vi "ControlApp.vi"() -> ()   [LabVIEW 2022 SP3]
uses:
  <vilib>/DAQmx/create/channels.llb/DAQmx Create Channel (AI-Voltage-Basic).vi
  <vilib>/DAQmx/create/channels.llb/DAQmx Create Channel (AO-Voltage-Basic).vi
  <vilib>/DAQmx/read.llb/DAQmx Read (Analog DBL 1Chan 1Samp).vi
  <vilib>/DAQmx/write.llb/DAQmx Write (Analog DBL 1Chan 1Samp).vi
  <vilib>/Simulation/Implementation/XNodeFramework/SimXNode/SimX.xnode
  SubVIs/Air Heater Model.vi
  <vilib>/Simulation/Implementation/Shared/SIMSCR Execution Mode.ctl
  <vilib>/Simulation/Scripting/Companion Diagram/SimConfigNode/_simSolvers.ctl
  <vilib>/Simulation/Scripting/Companion Diagram/SimConfigNode/SimParams.ctl
  <vilib>/Simulation/Scripting/Companion Diagram/SimConfigNode/SimDog.xnode
  <vilib>/OPCUA/controls/Write Status.ctl
  <vilib>/OPCUA/controls/NodeId.ctl
  <vilib>/OPCUA/client/Multiple Write Double.vi
  <vilib>/OPCUA/controls/OPC UA Client Refnum.ctl
panel:
  out "Status":bool
  out "OPC UA Client Reference":T1="tOPCUAClient3"
  out "Temperature":dbl=25.00772115553251 caption="Temperature [C]:" format="%.2g"
  out "Current Time":string="2018-10-12 13:37:48"
  out "Database Connection":refnum<k7>
  out "Error Out":errorcluster
  in  "Error In":errorcluster
  in  "Stop Button":bool
  in  "Start Button":bool
  in  "Tab Control":T2(tab)
  out "Measurement Chart":cluster{"Tout [C]":dbl, "Setpoint [C]":dbl}(graph)={"Tout [C]"=25.00772115553251, "Setpoint [C]"=25.0}
  out "Control Chart":dbl(graph)=1.0759899998167255
  in  "Process Type":enum16{"Model", "Real Process"}(ring)
  in  "Manual Control Signal [V]":dbl min=0.0 max=5.0 step=0.1 format="%.1g"
  in  "Auto?":bool=TRUE
  in  "Setpoint [C]":dbl(slide)=25.0 scale=20.0..50.0
  in  "PID Parameters":cluster{"Kp":dbl, "Ti [s]":dbl, "Td [s]":dbl}={"Kp"=0.55, "Ti [s]"=18.0, "Td [s]"=0.0}
  in  "Write to File":bool
  in  "File Path":path=path "C:/Temp/MeasurementData.lvm"
  in  "Write to SQL Server":bool
  in  "OPC Settings":T3={"OPC Server Endpoint URL"="opc.tcp://XPS15HPH:49580", "OPC Node Id"="ns=2;s=ProcessData.Temperature"}
  in  "Database":T4={"Data Source Name"="XPS15HPH\\SQLEXPRESS", "Database Name"="MEASUREMENTS", "User Name"="sa", "Password"="ullabella"} caption="Database Connection:"
  in  "DAQ Settings":T5={"Analog Input Channel"="Dev1/ai0", "AImin[V]"=1, "AImax[V]"=5, "Analog Output Channel"="Dev1/ao0", "AOmin[V]"=0, "AOmax[V]"=5} {"AOmax[V]" min=-10 max=10 step=1; "AOmin[V]" min=-10 max=10 step=1; "AImax[V]" min=-10 max=10 step=1; "AImin[V]" min=-10 max=10 step=1}
  out "Error Message":errorcluster
  in  "Exit Button":bool
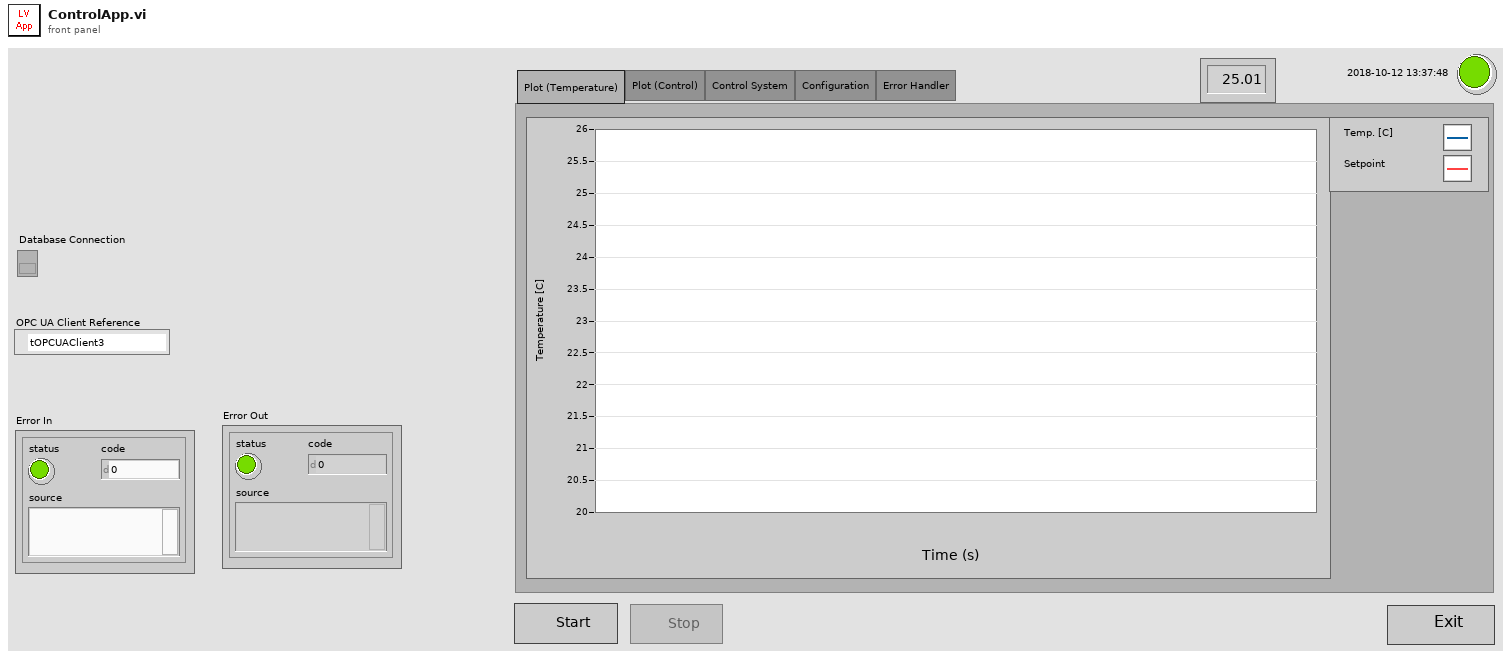
[diagram p1: front panel]
types:
  T1 = typedef "OPC UA Client Refnum.ctl" = refnum<k21>
  T2 = enum32{"Plot (Temperature)", "Plot (Control)", "Control System", "Configuration", "Error Handler", "Cloud Service"}
  T3 = cluster{"OPC Server Endpoint URL":string, "OPC Node Id":string}
  T4 = cluster{"Data Source Name":string, "Database Name":string, "User Name":string, "Password":string}
  T5 = cluster{"Analog Input Channel":tag, "AImin[V]":i32, "AImax[V]":i32, "Analog Output Channel":tag, "AOmin[V]":i32, "AOmax[V]":i32}
  T6 = enum8{"Enabled", "Disabled", "Disabled and Grayed Out"}
  T7 = enum16{"Simulate to Completion", "Single Time-Step Simulation (Fixed Step Only)"}
  T8 = typedef "SimParams.ctl" = cluster{"Initial Time (s)":dbl, "Final Time (s)":dbl, "Step Size (s)":dbl, "ODE Solver":T9, "Minimum Step Size (s)":dbl, "Maximum Step Size (s)":dbl, "Relative Tolerance":dbl, "Absolute Tolerance":dbl, "Software Timing":bool, "Initial Step Size (s)":dbl, "Automatic Fixed Step Size?":bool, "Automatic Discrete Step Size?":bool, "Discrete Step Size (s)":dbl, "Calculate using Time Step":bool, "Solver Wired?":bool, "Prev.Frm.Expected End":u64, "Prev.Frm.Actual End":u64, "Prev.Frm.Finished Late?":bool, "Prev.Iter.Expected End":u64, "Prev.Iter.Actual End":u64, "Prev.Iter.Finished Late?":bool, "Expected Iteration Start":u64, "Actual Iteration Start":u64, "Expected Frame Start":u64, "Actual Frame Start":u64, "Source Name":string, "Name":string, "Period":i64, "Deadline":i64, "Offset":i64, "Start":i64, "Priority":i32, "Timeout":i32, "Processor":i32, "Mode":enum32{"No Change", "Process missed periods, maintain original phase", "Discard missed periods, maintain original phase", "Process missed periods, ignore original phase", "Discard missed periods, ignore original phase"}, "Wakeup reason":enum32{"Normal", "Aborted", "Asynchronous wakeup", "Timing source error", "Timed loop error", "Timeout"}, "Error":errorcluster, "Source Type":string, "Secondary Source Type":string, "Global End Time":u64, "Global Start Time":u64, "Full Solver Reset":bool, "Execution Mode":T10, "Nan/Inf Check":bool, "Custom Solver Library":string, "Solver Is Variable":bool, "custom solver name":string, "Signal Collection Decimation":u32}
  T9 = typedef "_simSolvers.ctl" = enum16{"Runge-Kutta 1 (Euler)", "Runge-Kutta 2", "Runge-Kutta 3", "Runge-Kutta 4", "Runge-Kutta 23 (variable)", "Runge-Kutta 45 (variable)", "BDF (variable)", "Adams-Moulton (variable)", "Rosenbrock (variable)", "Discrete States Only", "SDIRK 4 (variable)", "Radau 5 (variable)", "Radau 9 (variable)", "Radau 13 (variable)", "Radau [Variable Order] (variable)", "Gear's Method (variable)", "Linearizer", "State Query", "Trim Eval", "Custom Solver"}
  T10 = typedef "SIMSCR Execution Mode.ctl" = enum16{"Simulate to Completion", "Single Time-Step Simulation (Fixed Step Only)"}
  T11 = cluster{"message mode":enum16{"None", "Sign", "Sign and Encrypt"}, "security":enum16{"Basic256", "Basic128Rsa15"}}
  T12 = cluster{"Vmin":dbl, "Vmax":dbl, "EUmin":dbl, "EUmax":dbl}
  T13 = typedef "NodeId.ctl" = string
  T14 = typedef "Write Status.ctl" = u32
  T15 = cluster{"node ID":T13, "value":dbl, "timestamp (current time)":timestamp, "node status":T14}
  T16 = cluster{"node ID":T13, "value":dbl, "timestamp (current time)":timestamp, "node status":T14}[]
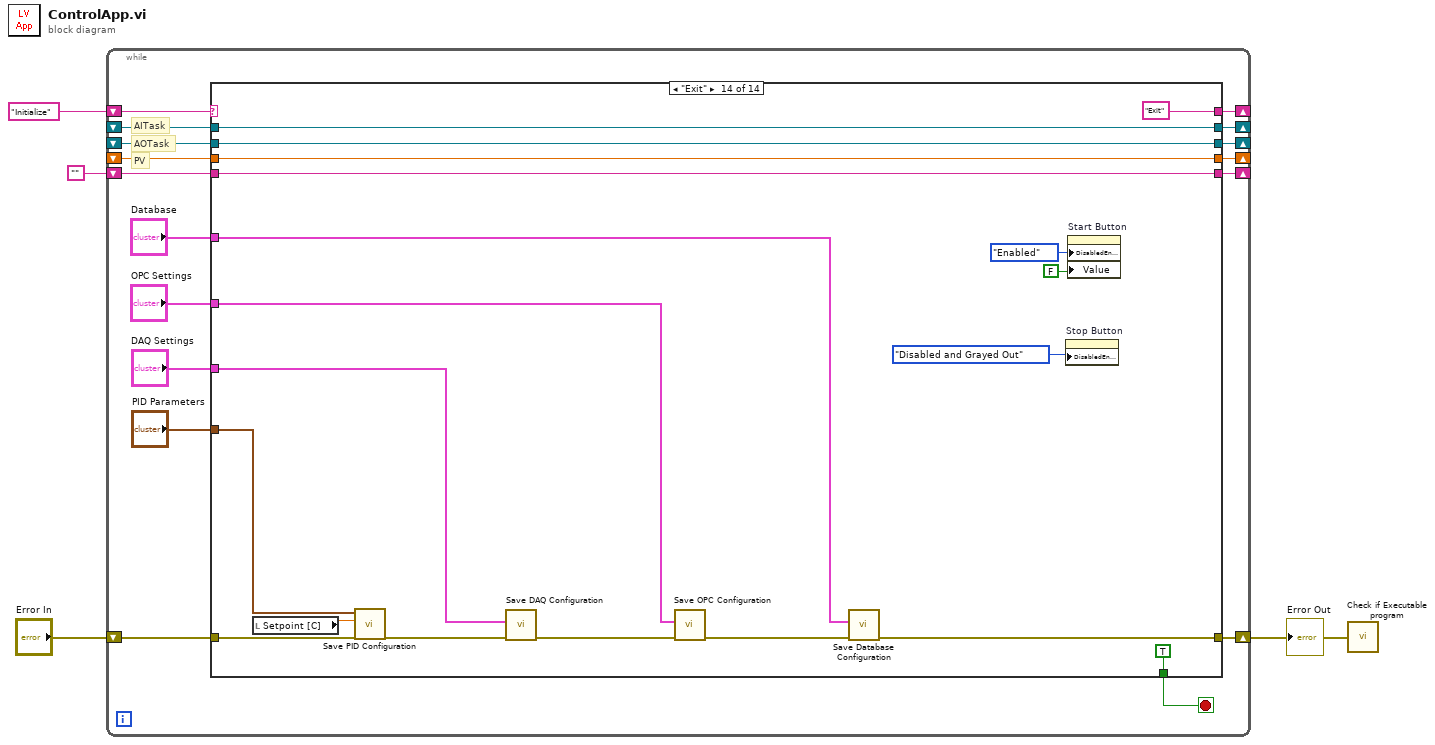
[diagram p0: block diagram]
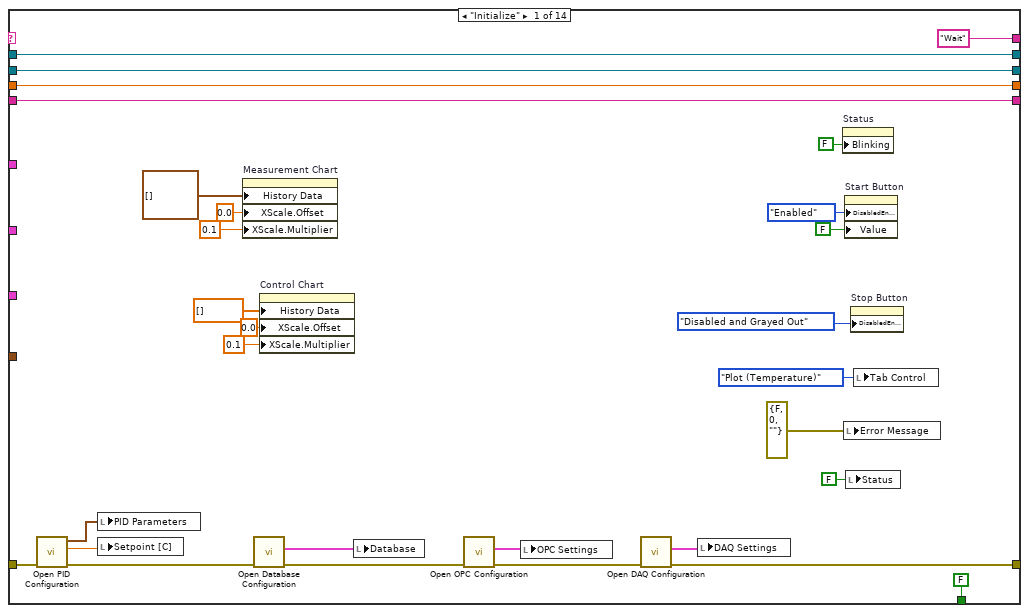
[diagram p2: hidden frame]
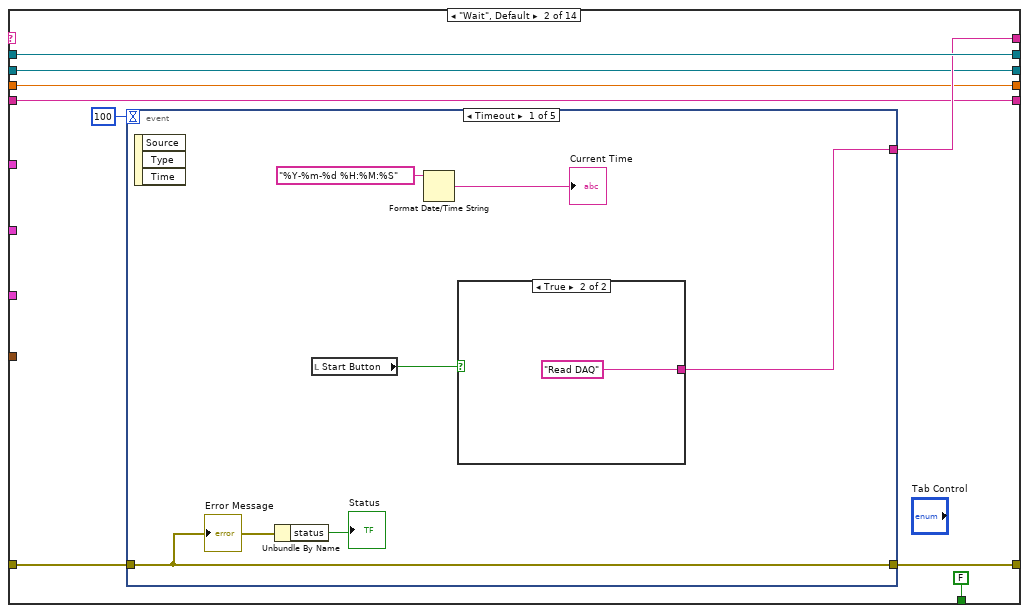
[diagram p3: hidden frame]
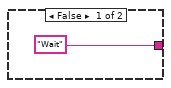
[diagram p4: hidden frame]
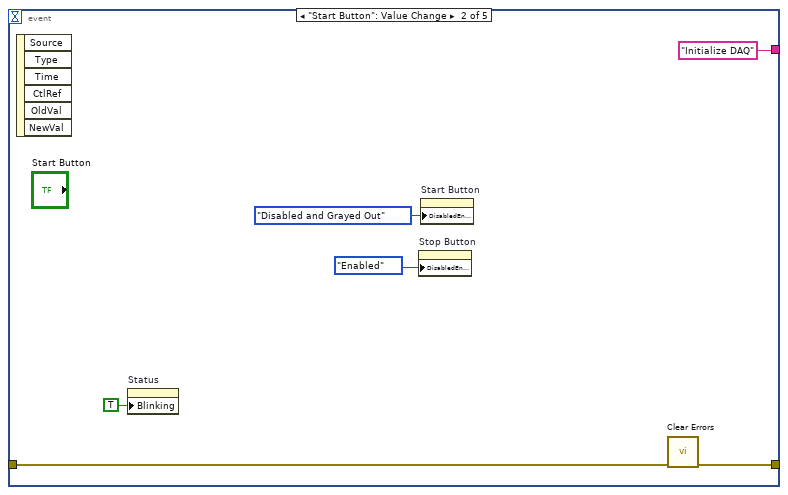
[diagram p5: hidden frame]
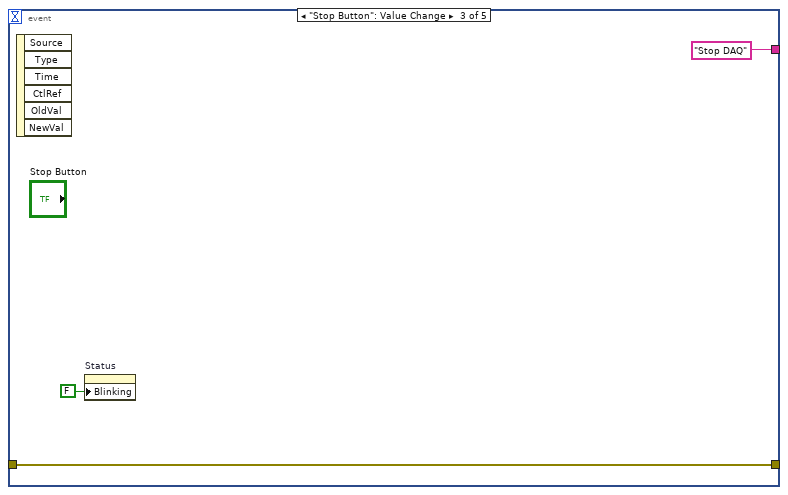
[diagram p6: hidden frame]
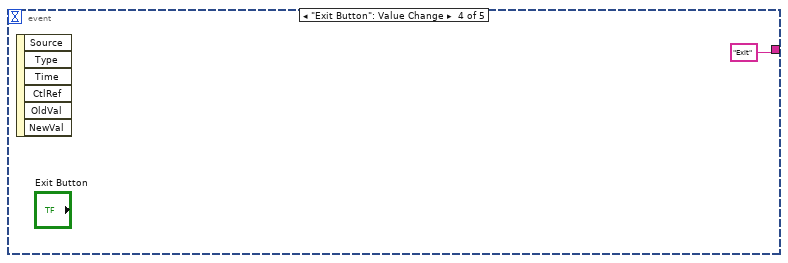
[diagram p7: hidden frame]
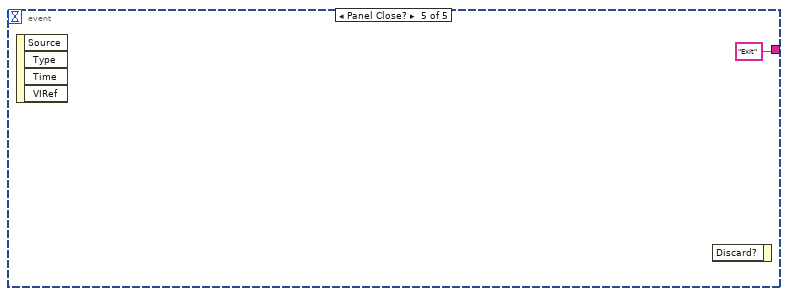
[diagram p8: hidden frame]
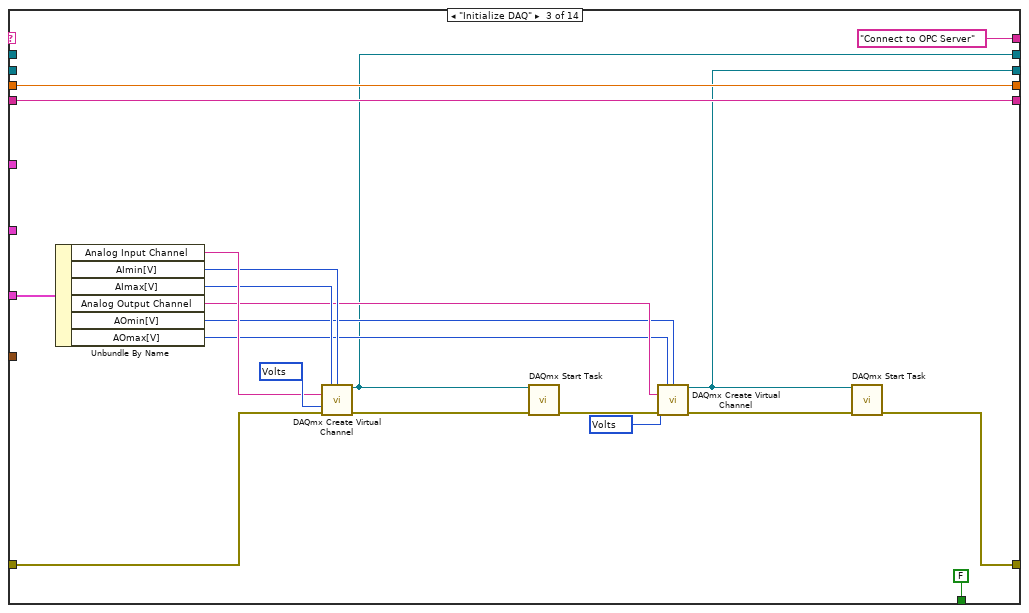
[diagram p9: hidden frame]
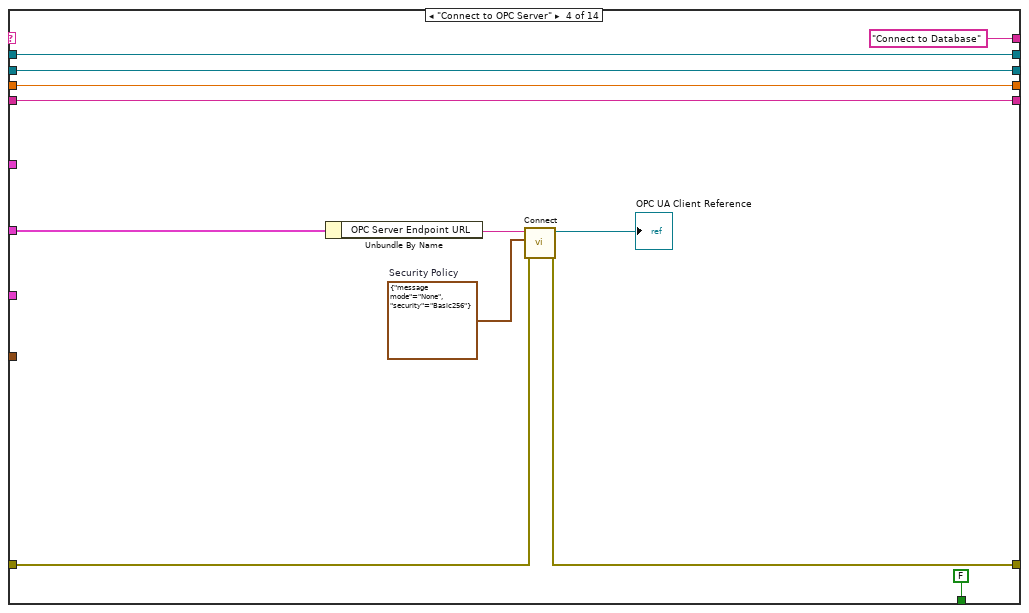
[diagram p10: hidden frame]
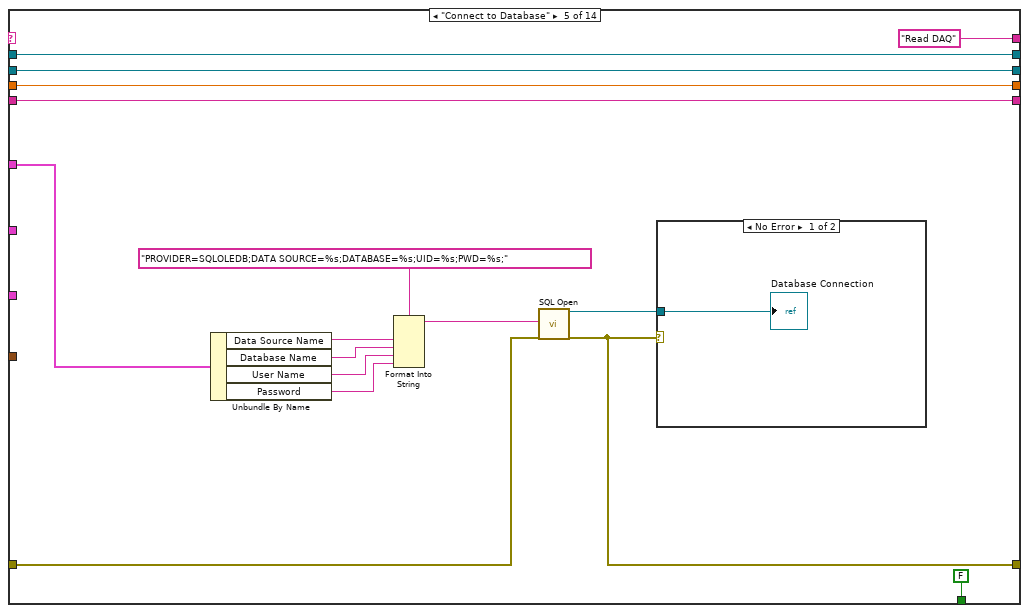
[diagram p11: hidden frame]
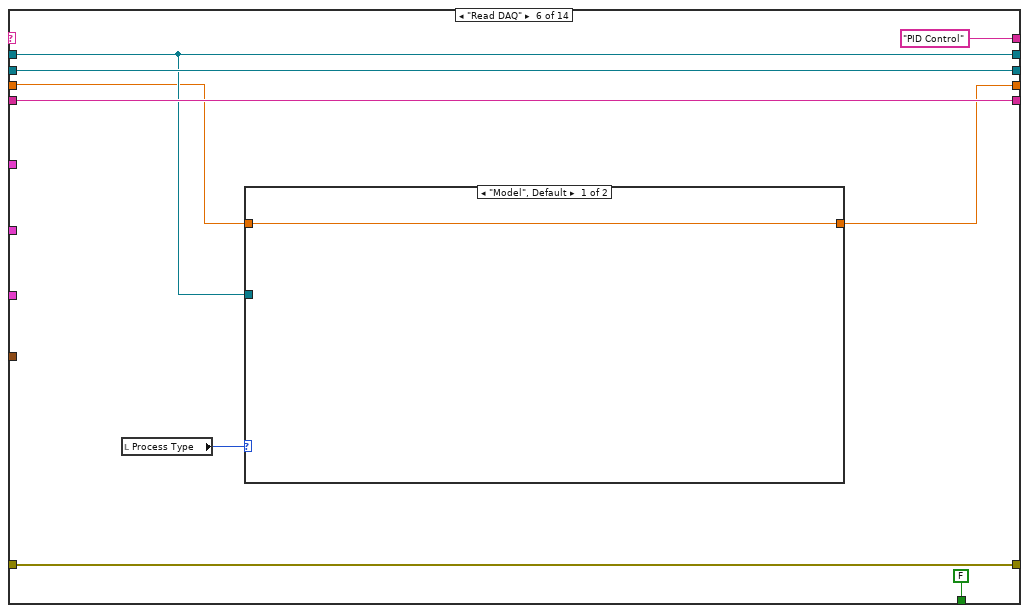
[diagram p13: hidden frame]
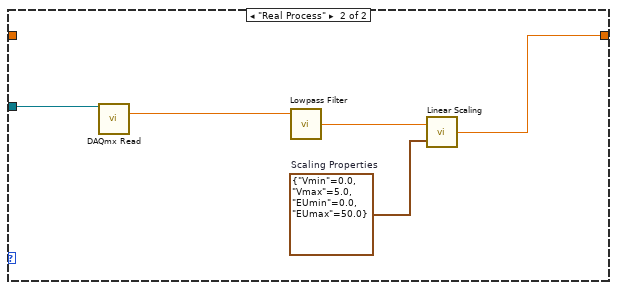
[diagram p14: hidden frame]
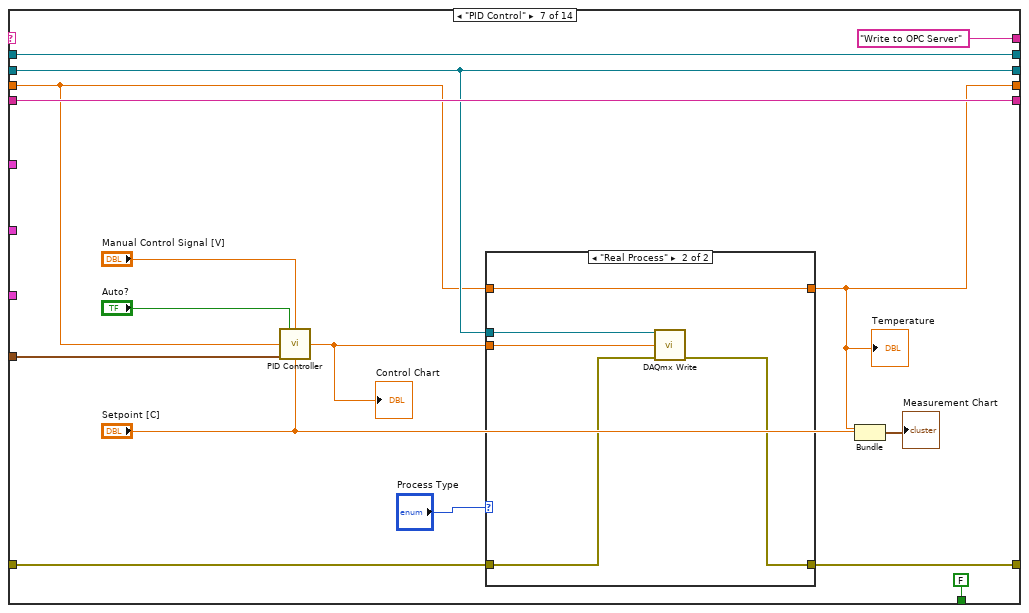
[diagram p15: hidden frame]
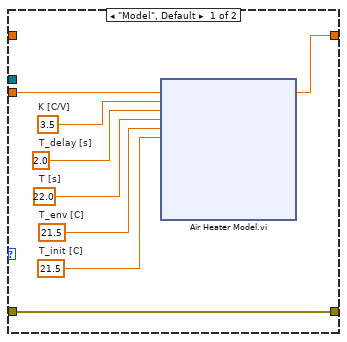
[diagram p16: hidden frame]
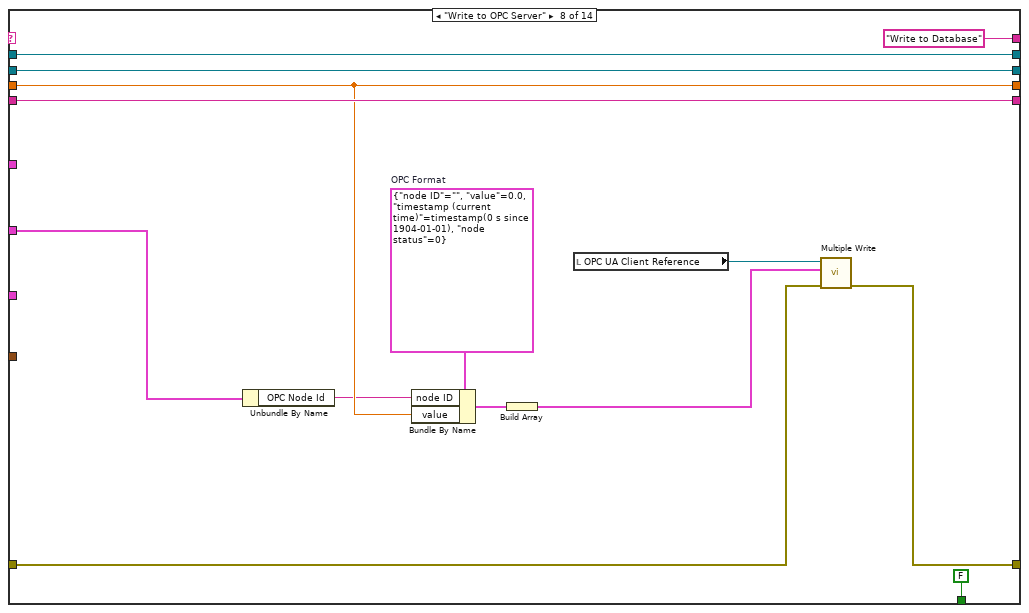
[diagram p17: hidden frame]
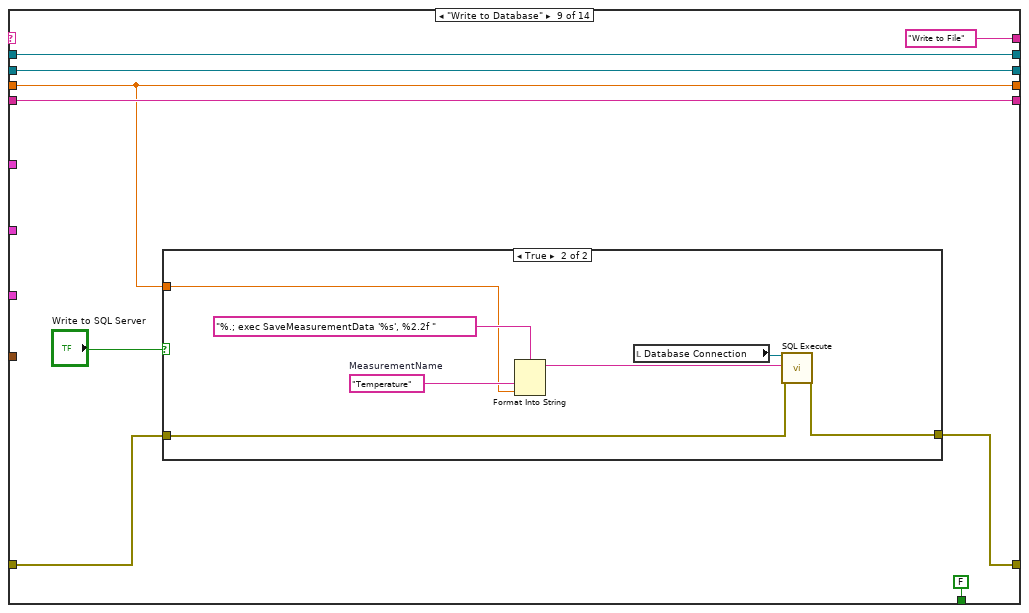
[diagram p18: hidden frame]
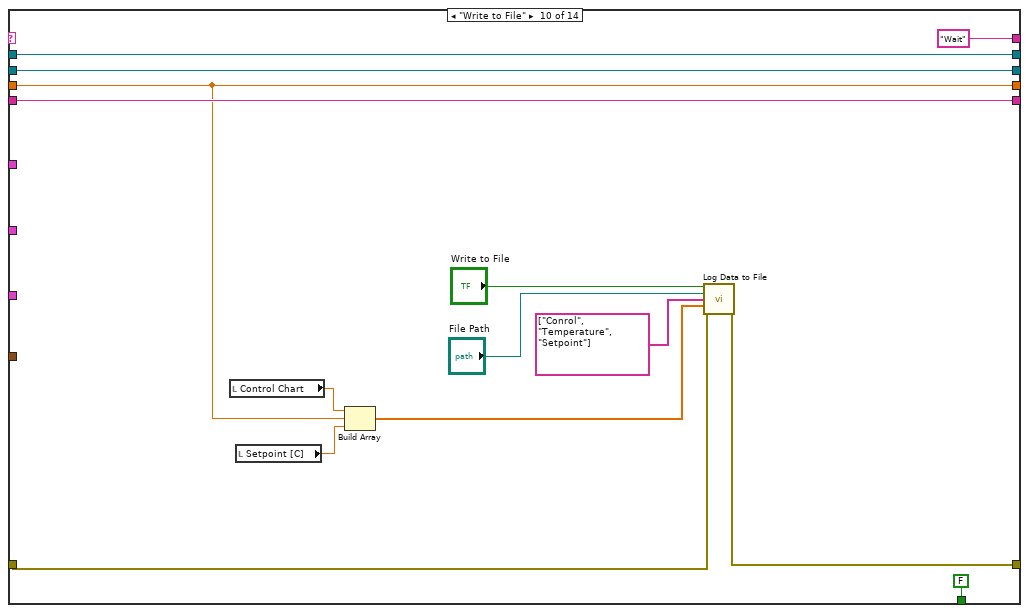
[diagram p20: hidden frame]
diagram:
  n1 = while {
    shift-right: [w20] -> _
    shift-left: "Initialize" -> [w21]
    shift-right: [w18] -> _
    shift-left: _ -> [w19]
    shift-right: [w15] -> _
    shift-left: _ -> [w16]
    shift-right: [w13] -> _
    shift-left: _ -> [w14]
    shift-right: [w11] -> _
    shift-left: "" -> [w12]
    shift-right: [w9] -> w1
    shift-left: "Error In" -> [w10]
    stop <- w17 stop-if-true
    # "PV"
    # "AOTask"
    # "AITask"
    n2 = case shown="\"Exit\"" w21 {
      tunnel: ["Wait" w57 "Connect to OPC Server" "Connect to Database" "Read DAQ" "PID Control" "Write to OPC Server" "Write to Database" "Write to File" "Wait" "Wait" "Wait" "Wait" "Exit"] -> w20
      tunnel: w19 -> [w49 w58 _ w110 w126 w129 w158 w221 w230 w252 w261 w273 w286 w305]
      tunnel: [w49 w58 w86 w110 w126 w129 w158 w221 w230 w252 w261 w273 w286 w305] -> w18
      tunnel: [FALSE FALSE FALSE FALSE FALSE FALSE FALSE FALSE FALSE FALSE FALSE FALSE FALSE TRUE] -> w17
      tunnel: w16 -> [w47 w55 _ w108 w124 w135 w150 w219 w228 w250 w258 w272 w284 w303]
      tunnel: [w47 w55 w82 w108 w124 w135 w150 w219 w228 w250 w258 w272 w284 w303] -> w15
      tunnel: w14 -> [w46 w54 w97 w107 w123 w128 w148 w211 w225 w246 w267 w276 w283 w302]
      tunnel: [w46 w54 w97 w107 w123 w131 w146 w211 w225 w246 w267 w276 w283 w302] -> w13
      tunnel: w12 -> [w45 w53 w96 w106 w122 w134 w156 w218 w227 w249 w266 w275 w282 w301]
      tunnel: [w45 w53 w96 w106 w122 w134 w156 w218 w227 w249 w266 w275 w282 w301] -> w11
      tunnel: w10 -> [w24 w51 w90 w102 w119 w132 w151 w214 w223 w240 w253 w270 w279 w288]
      tunnel: [w28 w52 w80 w103 w118 w132 w152 w215 w222 w239 w254 w271 w278 w293] -> w9
      tunnel: "Database" -> [_ _ _ _ w111 _ _ _ _ _ _ _ _ w296]
      tunnel: "OPC Settings" -> [_ _ _ w99 _ _ _ w208 _ _ _ _ _ w295]
      tunnel: "DAQ Settings" -> [_ _ w79 _ _ _ _ _ _ _ _ _ _ w292]
      tunnel: "PID Parameters" -> [_ _ _ _ _ _ w143 _ _ _ _ _ _ w290]
      frame "Initialize" {
        n3 = call "Open PID Configuration.vi"("Error In"=w24) -> ("Error Out"=w25:errorcluster, "SP"=w22:dbl, "PID Parameters"=w23:cluster{"Kp":dbl, "Ti [s]":dbl, "Td [s]":dbl})  [unwired: 8 in]
        n4 = local write "PID Parameters"(w23) -> ()
        n5 = local write "Setpoint [C]"(w22) -> ()
        n6 = property on="Measurement Chart" class="WFChart (strict)"("History Data"=cluster{"Tout [C]":dbl, "Setpoint [C]":dbl}[] [], "XScale.Offset"=0.0 ("X Scale.Offset and Multiplier:Offset"), "XScale.Multiplier"=0.1 ("X Scale.Offset and Multiplier:Multiplier")) -> ()  [unwired: 2 in, 2 out]
        n7 = call "Open Database Configuration.vi"("Error In"=w25) -> ("Error Out"=w31:errorcluster, "Database Connection"=w32:T4)  [unwired: 9 in]
        n8 = property on="Control Chart" class="WFChart (strict)"("History Data"=dbl[] [], "XScale.Offset"=0.0 ("X Scale.Offset and Multiplier:Offset"), "XScale.Multiplier"=0.1 ("X Scale.Offset and Multiplier:Multiplier")) -> ()  [unwired: 2 in, 2 out]
        n9 = local write "Database"(w32) -> ()
        n10 = call "Open OPC Configuration.vi"("Error In"=w31) -> ("Error Out"=w29:errorcluster, "OPC Settings"=w30:T3)  [unwired: 9 in]
        n11 = local write "OPC Settings"(w30) -> ()
        n12 = call "Open DAQ Configuration.vi"("Error In"=w29) -> ("Error Out"=w28:errorcluster, "DAQ Device Settings"=w27:T5)  [unwired: 9 in]
        n13 = local write "DAQ Settings"(w27) -> ()
        n14 = property on="Status" class="Bool (strict)"("Blinking"=FALSE) -> ()  [unwired: 2 in, 2 out]
        n15 = local write "Error Message"(errorcluster {"status"=FALSE, "code"=0, "source"=""} ("Error Message")) -> ()
        n16 = property on="Start Button" class="Bool (strict)"("DisabledEnum"=T6."Enabled" ("Disabled"), "Value"=FALSE ("Start DAQ Button")) -> ()  [unwired: 2 in, 2 out]
        n17 = local write "Status"(FALSE ("Status")) -> ()
        n18 = property on="Stop Button" class="Bool"("DisabledEnum"=T6."Disabled and Grayed Out" ("Disabled")) -> ()  [unwired: 2 in, 2 out]
        n19 = local write "Tab Control"(T2."Plot (Temperature)" ("Tab Control")) -> ()
      }
      frame "Wait", Default {
        n20 = event shown="[0] Timeout" {
          selector: _ -> [_ _ _ _ _]
          dyn-events: _ -> [_ _ _ _ _]
          timeout: 100 -> [_ _ _ _ _]
          tunnel: [w62 "Initialize DAQ" "Stop DAQ" "Exit" "Exit"] -> w57
          tunnel: w51 -> [w60 w70 w76 _ _]
          tunnel: [w60 w69 w76 _ _] -> w52
          event Timeout {
            n21 = event-data() -> ()  [unwired: 1 in, 3 out]
            n22 = Unbundle By Name(w60) -> ("status"=→"Status":bool)
            n23 = local read "Start Button"() -> (w63:bool)
            n24 = Format Date/Time String(time format string (%c)="%Y-%m-%d %H:%M:%S") -> (date/time string=→"Current Time":string)  [unwired: 2 in]
            n25 = case shown="True" w63 {
              tunnel: ["Wait" "Read DAQ"] -> w62
              frame False {
              }
              frame True {
              }
            }
            "Error Message" <- w60
          }
          event "Start Button": Value Change {
            n26 = event-data() -> ()  [unwired: 1 in, 6 out]
            n27 = property on="Status" class="Bool (strict)"("Blinking"=TRUE) -> ()  [unwired: 2 in, 2 out]
            n28 = property on="Stop Button" class="Bool"("DisabledEnum"=T6."Enabled" ("Disabled")) -> ()  [unwired: 2 in, 2 out]
            n29 = property on="Start Button" class="Bool (strict)"("DisabledEnum"=T6."Disabled and Grayed Out" ("Disabled")) -> ()  [unwired: 2 in, 2 out]
            n30 = call <vilib>:"Clear Errors.vi"("error in (no error)"=w70) -> ("error out"=w69:errorcluster)  [unwired: 5 in, 1 out]
          }
          event "Stop Button": Value Change {
            n31 = event-data() -> ()  [unwired: 1 in, 6 out]
            n32 = property on="Status" class="Bool (strict)"("Blinking"=FALSE) -> ()  [unwired: 2 in, 2 out]
          }
          event "Exit Button": Value Change {
            n33 = event-data() -> ()  [unwired: 1 in, 6 out]
          }
          event Panel Close? {
            n34 = event-data() -> ()  [unwired: 1 in, 4 out]
            n35 = event-data() -> ()  [unwired: 2 in, 1 out]
          }
        }
      }
      frame "Initialize DAQ" {
        w83 = 10348 items=["Volts"=10348, "From Custom Scale"=10065] ("units")
        w94 = 10348 items=["Volts"=10348, "From Custom Scale"=10065] ("units")
        n36 = Unbundle By Name(w79) -> ("Analog Input Channel"=w93:tag, "AImin[V]"=w91:i32, "AImax[V]"=w92:i32, "Analog Output Channel"=w89:tag, "AOmin[V]"=w88:i32, "AOmax[V]"=w87:i32)
        n37 = call-poly <vilib>:"DAQmx Create Virtual Channel.vi"("maximum value"=w92, "minimum value"=w91, "physical channels"=w93, "units"=w94, "error in"=w90) -> ("task out"=w86:refnum<k21>, "error out"=w85:errorcluster)  [unwired: 9 in]
        n38 = call <vilib>:"DAQmx Start Task.vi"("task/channels in"=w86, "error in"=w85) -> ("error out"=w84:errorcluster)  [unwired: 12 in, 1 out]
        n39 = call-poly <vilib>:"DAQmx Create Virtual Channel.vi"("maximum value"=w87, "minimum value"=w88, "physical channels"=w89, "units"=w83, "error in"=w84) -> ("task out"=w82:refnum<k21>, "error out"=w81:errorcluster)  [unwired: 9 in]
        n40 = call <vilib>:"DAQmx Start Task.vi"("task/channels in"=w82, "error in"=w81) -> ("error out"=w80:errorcluster)  [unwired: 12 in, 1 out]
      }
      frame "Connect to OPC Server" {
        w104 = T11 {"message mode"=enum."None", "security"=enum."Basic256"}  # Security Policy
        n41 = Unbundle By Name(w99) -> ("OPC Server Endpoint URL"=w100:string)
        n42 = call <vilib>:"Connect.vi"("error in (no error)"=w102, "security policy"=w104, "server endpoint URL"=w100) -> ("error out"=w103:errorcluster, "OPC UA client refnum out"=→"OPC UA Client Reference":T1)  [unwired: 6 in, 1 out]
      }
      frame "Connect to Database" {
        n43 = Unbundle By Name(w111) -> ("Data Source Name"=w115:string, "Database Name"=w114:string, "User Name"=w113:string, "Password"=w112:string)
        n44 = Format Into String(format string="PROVIDER=SQLOLEDB;DATA SOURCE=%s;DATABASE=%s;UID=%s;PWD=%s;", w115, w114, w113, w112) -> (resulting string=w116:string)  [unwired: 2 in, 1 out]
        n45 = call <vilib>:"SQL Open.vi"("ConnectionString In"=w116, "Error in (no error)"=w119) -> ("Connection Out"=w120:refnum<k7>, "Error out"=w118:errorcluster)  [unwired: 16 in]
        n46 = case shown="No Error" w118 {
          tunnel: w120 -> [w127 _]
          frame No Error {
            "Database Connection" <- w127
          }
          frame Error {
          }
        }
      }
      frame "Read DAQ" {
        n47 = local read "Process Type"() -> (w130:enum16{"Model", "Real Process"})
        n48 = case shown="\"Model\", Default" w130 {
          tunnel: [w137 w139] -> w131
          tunnel: w129 -> [_ w138]
          tunnel: w128 -> [w137 _]
          frame "Model", Default {
          }
          frame "Real Process" {
            w141 = T12 {"Vmin"=0.0, "Vmax"=5.0, "EUmin"=0.0, "EUmax"=50.0}  # Scaling Properties
            n49 = call-poly <vilib>:"DAQmx Read.vi"("task/channels in"=w138) -> ("data"=w140:dbl)  [unwired: 12 in, 2 out]
            n50 = call "Lowpass Filter.vi"("Filter Input"=w140) -> ("Filter Output"=w142:dbl)  [unwired: 2 in]
            n51 = call "Linear Scaling.vi"("Scaling Properties"=w141, "x"=w142) -> ("y"=w139:dbl)
          }
        }
      }
      frame "PID Control" {
        n52 = call "PID Controller.vi"("Auto?"="Auto?", "u_man [V]"="Manual Control Signal [V]", "Process Variable"=w148, "PID Parameters"=w143, "Setpoint [20-50deg]"="Setpoint [C]") -> ("u"=w147:dbl)  [unwired: 10 in]
        "Control Chart" <- w147
        n53 = case shown="\"Real Process\"" "Process Type" {
          tunnel: w147 -> [w165 w207]
          tunnel: [w166 w206] -> w152
          tunnel: w151 -> [w166 w205]
          tunnel: w150 -> [_ w204]
          tunnel: w148 -> [_ w203]
          tunnel: [w164 w203] -> w146
          frame "Model", Default {
            w159 = 21.5  # T_init [C]
            w160 = 21.5  # T_env [C]
            w161 = 22.0  # T [s]
            w162 = 2.0  # T_delay [s]
            w163 = 3.5  # K [C/V]
            n54 = xnode "Air Heater Model.vi"("u [V]"=w165, "K [C/V]"=w163, "T_delay [s]"=w162, "T [s]"=w161, "T_env [C]"=w160, "T_init [C]"=w159) -> ("Tout [C]"=w164:dbl)  [unwired: 2 in, 14 out]
          }
          frame "Real Process" {
            n55 = call-poly <vilib>:"DAQmx Write.vi"("task/channels in"=w204, "data"=w207, "error in"=w205) -> ("error out"=w206:errorcluster)  [unwired: 10 in, 2 out]
          }
        }
        "Temperature" <- w146
        n56 = Bundle("Tout [C]"=w146, "Setpoint [C]"="Setpoint [C]") -> (→"Measurement Chart":cluster{"Tout [C]":dbl, "Setpoint [C]":dbl})  [unwired: 1 in]
      }
      frame "Write to OPC Server" {
        w212 = T15 {"node ID"="", "value"=0.0, "timestamp (current time)"=timestamp(0 s since 1904-01-01), "node status"=0}  # OPC Format
        n57 = Unbundle By Name(w208) -> ("OPC Node Id"=w209:string)
        n58 = Bundle By Name(cluster=w212, "node ID"=w209, "value"=w211) -> (w213:T15)
        n59 = Build Array(w213) -> (w210:T16)
        n60 = local read "OPC UA Client Reference"() -> (w216:T1)
        n61 = call-poly <vilib>:"Multiple Write.vi"("error in (no error)"=w214, "requests"=w210, "OPC UA client refnum in"=w216) -> ("error out"=w215:errorcluster)  [unwired: 5 in, 3 out]
      }
      frame "Write to Database" {
        n62 = case shown="True" "Write to SQL Server" {
          tunnel: w225 -> [_ w234]
          tunnel: w223 -> [w231 w233]
          tunnel: [w231 w232] -> w222
          frame False {
          }
          frame True {
            w235 = "Temperature"  # MeasurementName
            n63 = Format Into String "Format Into String"(format string="%.; exec SaveMeasurementData '%s', %2.2f ", w235, w234) -> (resulting string=w237:string)  [unwired: 2 in, 1 out]
            n64 = local read "Database Connection"() -> (w236:refnum<k7>)
            n65 = call <vilib>:"SQL Execute.vi"("Connection In"=w236, "SQL Query"=w237, "Error in (no error)"=w233) -> ("Error out"=w232:errorcluster)  [unwired: 15 in, 1 out]
          }
        }
      }
      frame "Write to File" {
        n66 = local read "Control Chart"() -> (w247:dbl)
        n67 = local read "Setpoint [C]"() -> (w245:dbl)
        n68 = Build Array(w247, w246, w245) -> (w242:dbl[])
        n69 = call "Log Data to File.vi"("Logging Data to File"="Write to File", "File Path"="File Path", "Measurement Names"=string[] ["Conrol", "Temperature", "Setpoint"], "Data"=w242, "Error In"=w240) -> ("Error Out"=w239:errorcluster)  [unwired: 10 in]
      }
      frame "Stop DAQ" {
        n70 = call <vilib>:"DAQmx Stop Task.vi"("task/channels in"=w261, "error in"=w253) -> ("task out"=w260:refnum<k21>, "error out"=w257:errorcluster)  [unwired: 12 in]
        n71 = call <vilib>:"DAQmx Clear Task.vi"("task in"=w260, "error in"=w257) -> ("error out"=w256:errorcluster)  [unwired: 13 in]
        n72 = call <vilib>:"DAQmx Stop Task.vi"("task/channels in"=w258, "error in"=w256) -> ("task out"=w259:refnum<k21>, "error out"=w255:errorcluster)  [unwired: 12 in]
        n73 = call <vilib>:"DAQmx Clear Task.vi"("task in"=w259, "error in"=w255) -> ("error out"=w254:errorcluster)  [unwired: 13 in]
        n74 = property on="Stop Button" class="Bool"("DisabledEnum"=T6."Disabled and Grayed Out" ("Disabled")) -> ()  [unwired: 2 in, 2 out]
        n75 = property on="Start Button" class="Bool (strict)"("DisabledEnum"=T6."Enabled" ("Disabled"), "Value"=FALSE ("Start DAQ Button")) -> ()  [unwired: 2 in, 2 out]
      }
      frame "Disconnect OPC Server" {
        n76 = local read "OPC UA Client Reference"() -> (w269:T1)
        n77 = call <vilib>:"Disconnect.vi"("error in (no error)"=w270, "OPC UA client refnum in"=w269) -> ("error out"=w271:errorcluster)  [unwired: 9 in]
      }
      frame "Disconnect from Database" {
        n78 = local read "Database Connection"() -> (w280:refnum<k7>)
        n79 = call <vilib>:"SQL Close.vi"("Connection In"=w280, "Error in (no error)"=w279) -> ("Error out"=w278:errorcluster)  [unwired: 17 in]
      }
      frame "Exit" {
        n80 = local read "Setpoint [C]"() -> (w287:dbl)
        n81 = call "Save PID Configuration.vi"("Error In"=w288, "SP"=w287, "PID Parameters"=w290) -> ("Error Out"=w289:errorcluster)  [unwired: 8 in]
        n82 = call "Save DAQ Configuration.vi"("Error In"=w289, "DAQ Device Settings"=w292) -> ("Error Out"=w291:errorcluster)  [unwired: 9 in]
        n83 = call "Save OPC Configuration.vi"("Error In"=w291, "OPC Settings"=w295) -> ("Error Out"=w294:errorcluster)  [unwired: 9 in]
        n84 = call "Save Database Configuration.vi"("Error In"=w294, "Database Connection"=w296) -> ("Error Out"=w293:errorcluster)  [unwired: 9 in]
        n85 = property on="Stop Button" class="Bool"("DisabledEnum"=T6."Disabled and Grayed Out" ("Disabled")) -> ()  [unwired: 2 in, 2 out]
        n86 = property on="Start Button" class="Bool (strict)"("DisabledEnum"=T6."Enabled" ("Disabled"), "Value"=FALSE ("Start DAQ Button")) -> ()  [unwired: 2 in, 2 out]
      }
    }
  }
  "Error Out" <- w1
  n87 = call "Check if Executable program.vi"("error in (no error)"=w1) -> ()  [unwired: 1 out]
